vi "ServerCommsCheck.vi"() -> (0 "ServerUp?":bool)   [LabVIEW 2018]
uses:
  Anemometry/Anemometry Sub Vis/Controls/App_Global.ctl
  Anemometry/Anemometry Sub Vis/Globals/Dynamic_call_global.ph.vi
  Anemometry/Anemometry Sub Vis/Globals/Constants_global.vi
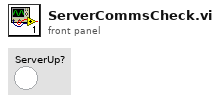
[diagram p1: front panel]
types:
  T1 = typedef "App_Global.ctl" = enum16{"Read Global", "Write to Global", "Initialise Array"}
  T2 = enum32{"Bad", "Idle", "Run top level", "Running"}
  T3 = typedef "App_Ref_Cluster.ctl" = cluster{"Server IP & Port No":string, "Application reference":refnum<vi>}
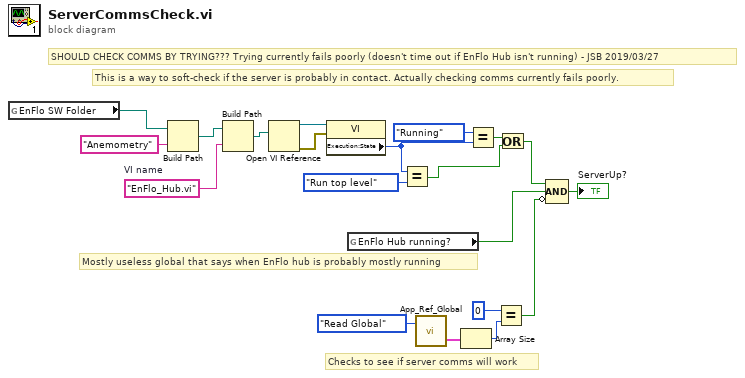
[diagram p0: block diagram]
diagram:
  w12 = "EnFlo_Hub.vi"  # VI name
  # "This is a way to soft-check if the server is probably in contact. Actually checking comms currently fails poorly."
  # "SHOULD CHECK COMMS BY TRYING??? Trying currently fails poorly (doesn't time out if EnFlo Hub isn't running) - JSB 2019/03/27"
  # "Mostly useless global that says when EnFlo hub is probably mostly running"
  # "Checks to see if server comms will work"
  n1 = global read "Constants_global.vi" "EnFlo SW Folder"() -> (w4:path)
  n2 = Build Path(base path=w4, name or relative path="Anemometry") -> (appended path=w3:path)
  n3 = Build Path(base path=w3, name or relative path=w12) -> (appended path=w18:path)
  n4 = Open VI Reference(vi path=w18) -> (vi reference=w16:refnum<vi>, error out=w17:errorcluster)  [unwired: 2 in, 3 out]
  n5 = property class="VI"(reference=w16, error in=w17) -> ("Execution:State"=w15:T2)  [unwired: 2 out]
  n6 = global read "Dynamic_call_global.ph.vi" "EnFlo Hub running?"() -> (w10:bool)
  n7 = Equal?(x=w15, y=T2."Run top level" ("Execution:State")) -> (x = y?=w13:bool)
  n8 = call "App_Ref_Global.vi"("Mode"=App_Global."Read Global") -> ("Output Array"=w8:T3[])  [unwired: 2 in]
  n9 = Array Size(array=w8) -> (size(s)=w7:i32)
  n10 = Equal?(x=T2."Running" ("Execution:State"), y=w15) -> (x = y?=w14:bool)
  n11 = Equal?(x=0, y=w7) -> (x = y?=w5:bool)
  n12 = Or(x=w14, y=w13) -> (x .or. y?=w11:bool)
  n13 = Compound Arithmetic op=AND(w11, w10, invert w5) -> (→"ServerUp?":bool)
